vi "globalSetUp.vi"(8 "error in (no error)":errorcluster, 11 "testcase-CSMStatus in":refnum<class "testcase-CSMBroadcast.lvclass">) -> (0 "error out":errorcluster, 3 "testcase-CSMStatus out":refnum<class "testcase-CSMBroadcast.lvclass">)   [LabVIEW 2017, in "testcase-CSMBroadcast.lvclass"]
uses:
  testcase-CSMBroadcast.lvclass
  <vilib>/addons/_JKI Toolkits/VI Tester/TestCase.llb/TestCase.lvclass
  CSM/CSM-Testcase.lvlib
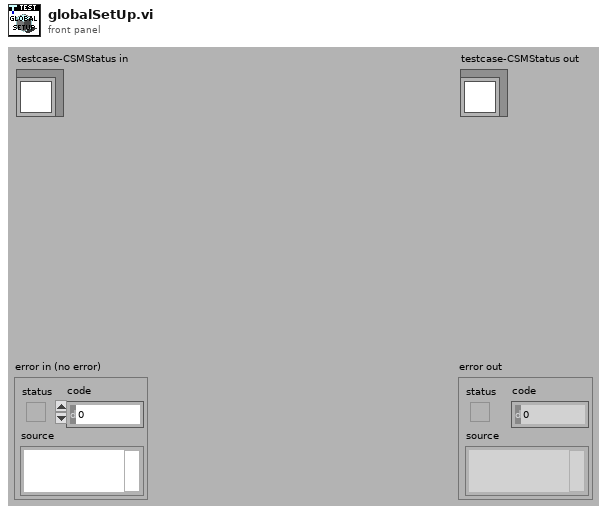
[diagram p1: front panel]
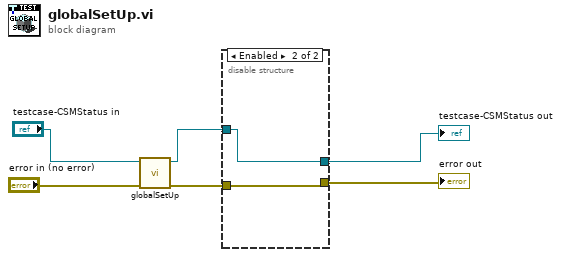
[diagram p0: block diagram]
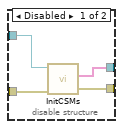
[diagram p2: hidden frame]
diagram:
  n1 = call-parent "globalSetUp.vi"("error in (no error)"="error in (no error)", "TestCase in"="testcase-CSMStatus in") -> ("error out"=w3:errorcluster, "TestCase out"=w1:refnum<class "testcase-CSMBroadcast.lvclass">)  [unwired: 8 in]
  n2 = disable-structure shown="Enabled" {
    disable-tunnel: w3 -> [w10 w11]
    disable-tunnel: [w9 w11] -> w6
    disable-tunnel: w1 -> [w8 w12]
    disable-tunnel: [w7 w12] -> w5
    frame Disabled {
      n3 = call "InitCSMs.vi"("error in"=w10, 11:w8) -> ("error out"=w9:errorcluster, "CSMs"=w7:string[])  [unwired: 8 in]
    }
    frame Enabled {
    }
  }
  "error out" <- w6
  "testcase-CSMStatus out" <- w5
